vi "Update Entity Status.vi"(7 "entity type":i32, 8 "error in (no error)":errorcluster, 9 "Status":string, 10 "Enqueuer":refnum<class "Message Enqueuer.lvclass">, 11 "entities in":refnum<class "Entity Table.lvclass">) -> (0 "error out":errorcluster, 3 "entities out":refnum<class "Entity Table.lvclass">)   [LabVIEW 2023, in "Entity Table.lvclass"]
doc: "Search for an entity by enqueuer refnum in the appropriate table and update its details if found."
uses:
  Entity Table.lvclass
  <vilib>/ActorFramework/Message Enqueuer/Message Enqueuer.lvclass
  Entity Table.lvclass/Entity Table.ctl
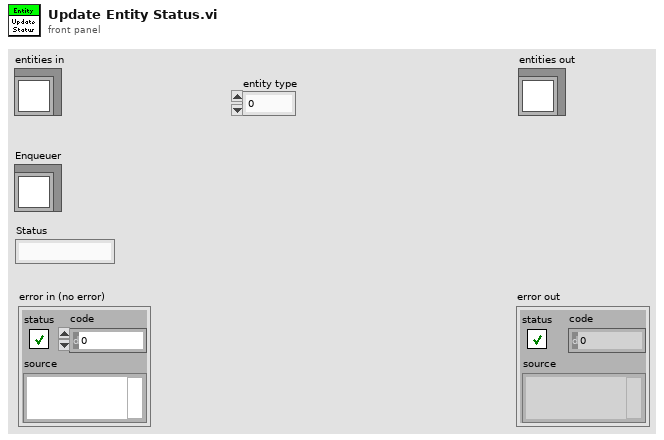
[diagram p1: front panel]
types:
  T1 = typedef "Entity Table.lvclass/Entity Table Element.ctl" = cluster{"Entity":refnum<class "Message Enqueuer.lvclass">[], "Entity Data":T2[]}
  T2 = typedef "Entity Table.lvclass/Entity Data.ctl" = cluster{"Name":string, "Status":string}
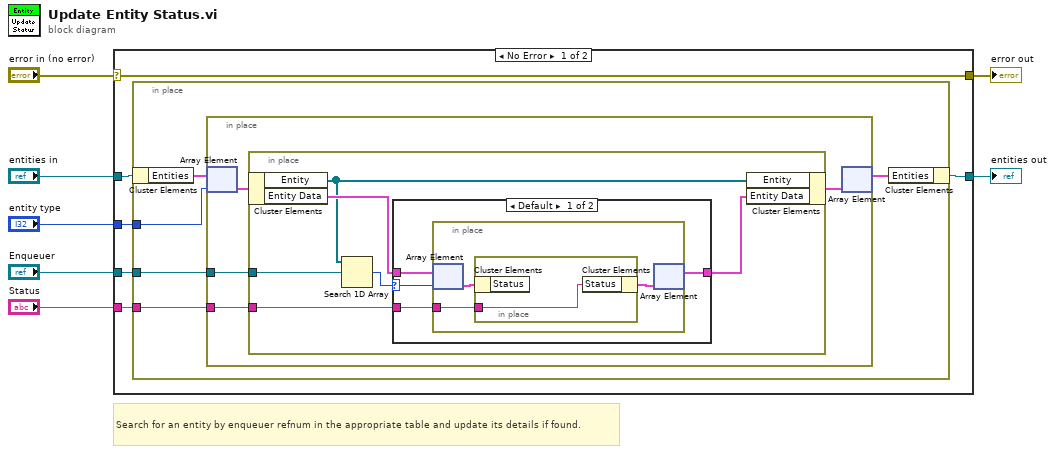
[diagram p0: block diagram]
diagram:
  # "Search for an entity by enqueuer refnum in the appropriate table and update its details if found."
  n1 = case shown="No Error" "error in (no error)" {
    selector: "error in (no error)" -> [w11 w39]
    tunnel: [w11 w39] -> w6
    tunnel: "entities in" -> [w9 w38]
    tunnel: [w8 w38] -> w4
    tunnel: "entity type" -> [w13 _]
    tunnel: "Enqueuer" -> [w12 _]
    tunnel: "Status" -> [w10 _]
    frame No Error {
      n2 = in-place "In Place Element Structure" {
        in-place-border: w13 -> [w18]
        in-place-border: w12 -> [w17]
        in-place-border: w10 -> [w16]
        n3 = in-place-cluster #1 ("Unbundle / Bundle Elements")(w9) -> ("Entities"=w15:T1[])
        n4 = in-place "In Place Element Structure" {
          in-place-border: w17 -> [w21]
          in-place-border: w16 -> [w19]
          n5 = in-place-array #2 ("Array Index / Replace Elements")(w15, w18) -> (w22:T1)
          n6 = in-place "In Place Element Structure" {
            in-place-border: w21 -> [w28]
            in-place-border: w19 -> [w23]
            n7 = in-place-cluster #3 ("Unbundle / Bundle Elements")(w22) -> ("Entity"=w24:refnum<class "Message Enqueuer.lvclass">[], "Entity Data"=w26:T2[])
            n8 = Search 1D Array(1D array=w24, element=w28) -> (index of element=w27:i32)  [unwired: 1 in]
            n9 = case shown="Default" w27 {
              selector: w27 -> [w31 _]
              tunnel: w26 -> [w32 w37]
              tunnel: [w30 w37] -> w25
              tunnel: w23 -> [w29 _]
              frame Default {
                n10 = in-place "In Place Element Structure" {
                  in-place-border: w29 -> [w33]
                  n11 = in-place-array #4 ("Array Index / Replace Elements")(w32, w31) -> (w35:T2)
                  n12 = in-place "In Place Element Structure" {
                    in-place-border: w33 -> [w36]
                    n13 = in-place-cluster #5 ("Unbundle / Bundle Elements")(w35) -> ()  [unwired: 1 out]
                    n14 = in-place-cluster #5 ("Unbundle / Bundle Elements")("Status"=w36) -> (w34:T2)
                  }
                  n15 = in-place-array #4 ("Array Index / Replace Elements")(w34) -> (w30:T2[])  [unwired: 1 out]
                }
              }
              frame -1 {
                # "No match found."
              }
            }
            n16 = in-place-cluster #3 ("Unbundle / Bundle Elements")("Entity"=w24, "Entity Data"=w25) -> (w20:T1)
          }
          n17 = in-place-array #2 ("Array Index / Replace Elements")(w20) -> (w14:T1[])  [unwired: 1 out]
        }
        n18 = in-place-cluster #1 ("Unbundle / Bundle Elements")("Entities"=w14) -> (w8:refnum<class "Entity Table.lvclass">)
      }
    }
    frame Error {
    }
  }
  "error out" <- w6
  "entities out" <- w4
